vi "Data_Base_logging.vi"() -> (1 "Logging On?":bool, 2 "Close Loop with Pitot?":bool, 3 "Rig Name":string, 4 "DB Setup files":string[](array[string])=["EnFlo_Tunnel DB setup.xls", "A_Tunnel DB setup.xls", "D_Tunnel DB setup.xls", "Aero_Tunnel DB setup.xls", "CPP_Tunnel1 DB setup.xls", "CPP_Tunnel2 DB setup.xls", "CPP_Tunnel3 DB setup.xls"] caption="DB Setup files (from EnFlo Tun Setup Global)")   [LabVIEW 2013]
uses:
  Controls/Server_Comms.ctl
  Globals/Preference_global.vi
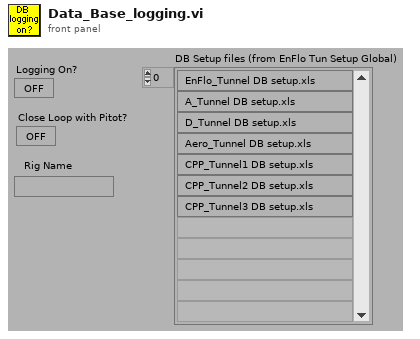
[diagram p1: front panel]
types:
  T1 = typedef "Server_Comms.ctl" = enum16{"Server Link Healthy", "Do Not Link To Server"}
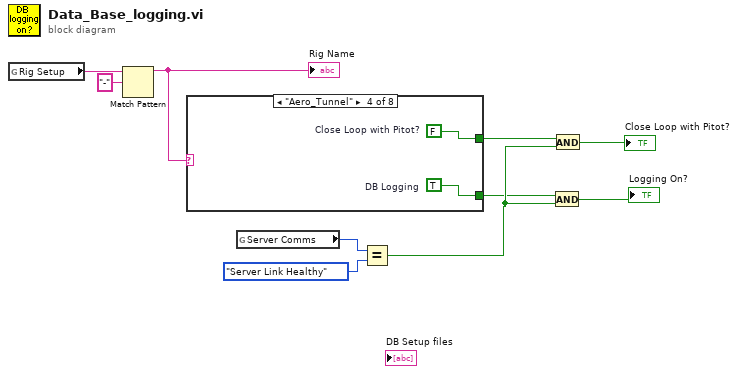
[diagram p0: block diagram]
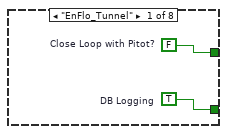
[diagram p2: hidden frame]
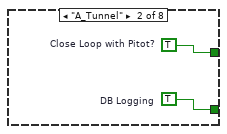
[diagram p3: hidden frame]
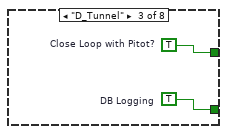
[diagram p4: hidden frame]
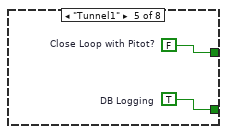
[diagram p5: hidden frame]
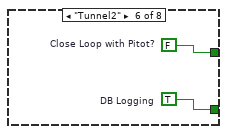
[diagram p6: hidden frame]
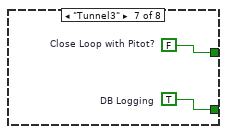
[diagram p7: hidden frame]
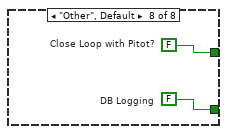
[diagram p8: hidden frame]
diagram:
  n1 = global read "Preference_global.vi" "Rig Setup"() -> (w3:string)
  n2 = Match Pattern(string=w3, regular expression="-") -> (before substring=w1:string)  [unwired: 4 out]
  "Rig Name" <- w1
  n3 = case shown="\"Aero_Tunnel\"" w1 {
    tunnel: [w12 w14 w16 w18 w20 w22 w24 w26] -> w5
    tunnel: [w11 w13 w15 w17 w19 w21 w23 w25] -> w4
    frame "EnFlo_Tunnel" {
      w11 = TRUE  # DB Logging
      w12 = FALSE  # Close Loop with Pitot?
    }
    frame "A_Tunnel" {
      w13 = TRUE  # DB Logging
      w14 = TRUE  # Close Loop with Pitot?
    }
    frame "D_Tunnel" {
      w15 = TRUE  # DB Logging
      w16 = TRUE  # Close Loop with Pitot?
    }
    frame "Aero_Tunnel" {
      w17 = TRUE  # DB Logging
      w18 = FALSE  # Close Loop with Pitot?
    }
    frame "Tunnel1" {
      w19 = TRUE  # DB Logging
      w20 = FALSE  # Close Loop with Pitot?
    }
    frame "Tunnel2" {
      w21 = TRUE  # DB Logging
      w22 = FALSE  # Close Loop with Pitot?
    }
    frame "Tunnel3" {
      w23 = TRUE  # DB Logging
      w24 = FALSE  # Close Loop with Pitot?
    }
    frame "Other", Default {
      w25 = FALSE  # DB Logging
      w26 = FALSE  # Close Loop with Pitot?
    }
  }
  n4 = global read "Preference_global.vi" "Server Comms"() -> (w9:T1)
  n5 = Equal?(x=w9, y=Server_Comms."Server Link Healthy" ("Server Comms")) -> (x = y?=w6:bool)
  n6 = And(x=w4, y=w6) -> (x .and. y?=→"Logging On?":bool)
  n7 = And(x=w5, y=w6) -> (x .and. y?=→"Close Loop with Pitot?":bool)
